vi "Receive (with Error In).vi"(8 "error in (no error)":errorcluster, 9 "timeout in ms (5000)":i32=5000, 11 "MGR in":refnum<class "MGR (Receive type).lvclass">) -> (0 "error out":errorcluster, 1 "Label":string, 2 "Message":refnum<class "MSG.lvclass">, 3 "MGR out":refnum<class "MGR (Receive type).lvclass">)   [LabVIEW 2011, in "Messenging.lvlib" / "MGR (Receive type).lvclass"]
uses:
  MGR (Receive type).lvclass
  ErrorMessage/ErrorMessage.lvclass
  TextVarientMessage/MSG.lvclass
panel:
  # "MSRReceiveTimedOut"
  # "MSRReceiverError"
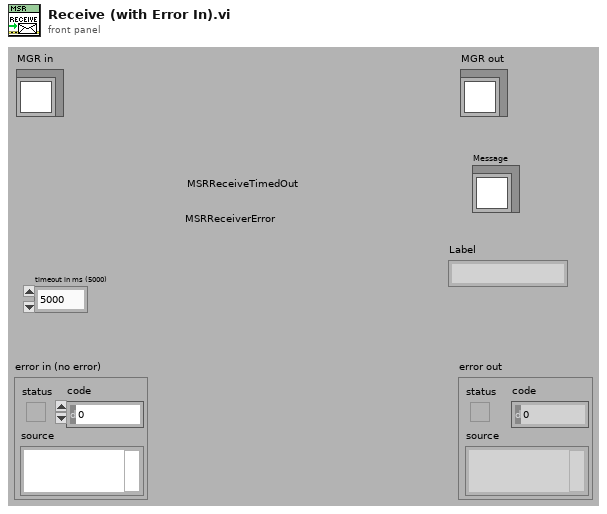
[diagram p1: front panel]
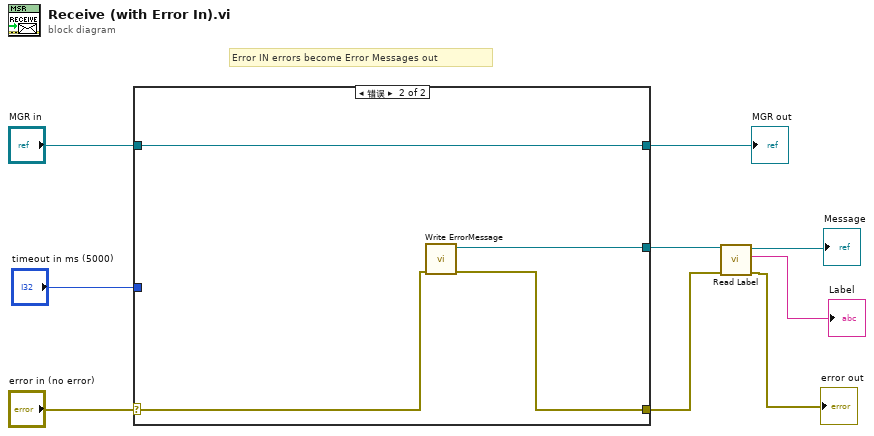
[diagram p0: block diagram]
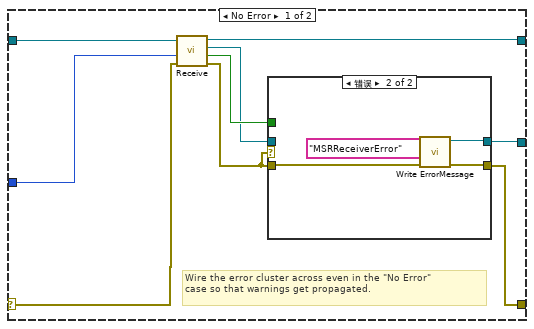
[diagram p2: hidden frame]
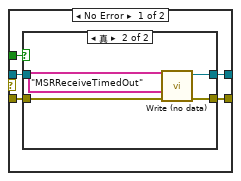
[diagram p3: hidden frame]
diagram:
  # "Error IN errors become Error Messages out"
  n1 = case shown="错误" "error in (no error)" {
    selector: "error in (no error)" -> [w15 w34]
    tunnel: [w11 w35] -> w2
    tunnel: [w17 w37] -> w7
    tunnel: "MGR in" -> [w18 w37]
    tunnel: "timeout in ms (5000)" -> [w16 _]
    tunnel: [w12 w36] -> w5
    frame No Error {
      # "Wire the error cluster across even in the \"No Error\"\ncase so that warnings get propagated."
      n2 = call-dynamic "Receive.vi"("error in (no error)"=w15, "timeout in ms (-1)"=w16, "Messenger in"=w18) -> ("error out"=w10:errorcluster, "timed out?"=w14:bool, "Message"=w13:refnum<class "MSG.lvclass">, "Messenger out"=w17:refnum<class "MGR (Receive type).lvclass">)  [unwired: 5 out]
      n3 = case shown="错误" w10 {
        tunnel: w14 -> [w23 _]
        tunnel: w13 -> [w22 _]
        tunnel: w10 -> [w21 w31]
        tunnel: [w20 w32] -> w12
        tunnel: [w19 w33] -> w11
        frame No Error {
          n4 = case shown="真" w23 {
            tunnel: [w25 w28] -> w20
            tunnel: w22 -> [w25 _]
            tunnel: w21 -> [w24 w27]
            tunnel: [w24 w26] -> w19
            frame False {
            }
            frame True {
              n5 = call "Write (no data).vi"("error in (no error)"=w27, "Label"="MSRReceiveTimedOut" ("Text")) -> ("error out"=w26:errorcluster, "Message"=w28:refnum<class "MSG.lvclass">)  [unwired: 8 out]
            }
          }
        }
        frame Error {
          n6 = call "Write ErrorMessage.vi"("error (to be sent)"=w31, "Label"="MSRReceiverError") -> ("error out"=w33:errorcluster, "Message"=w32:refnum<class "ErrorMessage.lvclass">)  [unwired: 1 in, 7 out]
        }
      }
    }
    frame Error {
      n7 = call "Write ErrorMessage.vi"("error (to be sent)"=w34) -> ("error out"=w35:errorcluster, "Message"=w36:refnum<class "ErrorMessage.lvclass">)  [unwired: 2 in, 7 out]
    }
  }
  "MGR out" <- w7
  n8 = call-dynamic "Read Label.vi"("error in (no error)"=w2, "Message"=w5) -> ("error out"=→"error out":errorcluster, "Label"=→"Label":string, "Message"=→"Message":refnum<class "MSG.lvclass">)  [unwired: 7 out]
